vi "Error Handler - Event Handling Loop.vi"(8 "error in (no error)":errorcluster, 10 "Ignore Errors (Runtime)":i32[](array[numeric])) -> (0 "dup error in":errorcluster, 3 "channel":T1)   [LabVIEW 2019]
doc: "Process an error that occurred in the Event Handling Loop, either by ignoring it, or generating an \"Error\" message."
uses:
  Message Queue/Message Cluster.ctl
  03.3 Queued Message Handler/support/Message Queue/Message Queue.lvlib
  <extravilib>/ChannelInstances/Messenger-t'Message Queue.lvlib-Message Cluster.ctl'/))Channel.ctl
  <extravilib>/ChannelInstances/Messenger-t'Message Queue.lvlib-Message Cluster.ctl'.lvlib
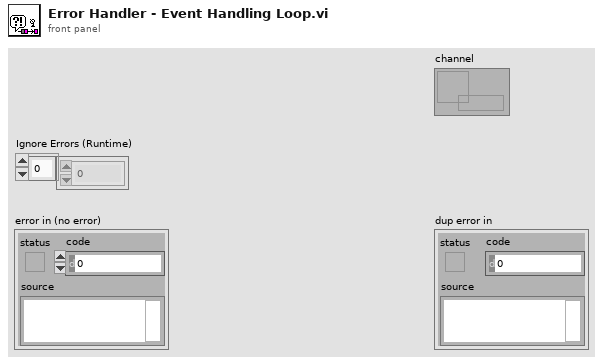
[diagram p1: front panel]
types:
  T1 = typedef "Messenger-t'Message Queue.lvlib-Message Cluster.ctl'.lvlib/))Channel.ctl" = refnum<queue>
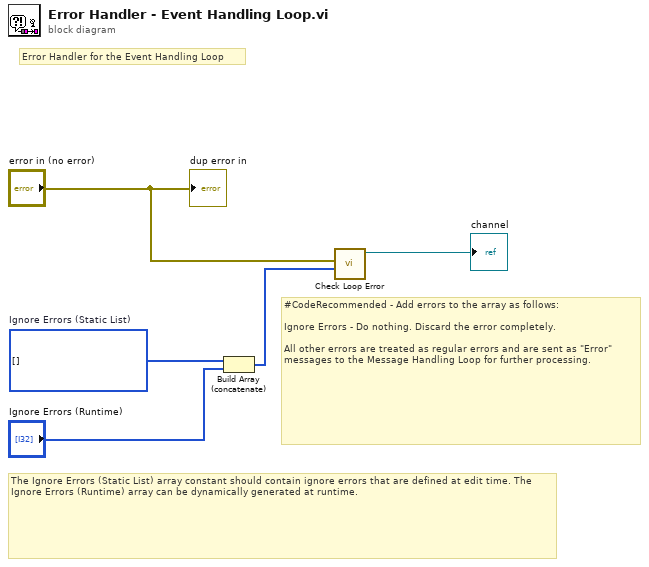
[diagram p0: block diagram]
diagram:
  w5 = i32[] []  # Ignore Errors (Static List)
  # "The Ignore Errors (Static List) array constant should contain ignore errors that are defined at edit time. The Ignore Errors (Runtime) array can be dynamically generated at runtime."
  # "#CodeRecommended - Add errors to the array as follows:\n\nIgnore Errors - Do nothing. Discard the error completely.\n\nAll other errors are treated as regular errors and are sent as \"Error\" messages to the Message Handling Loop for further processing."
  # "Error Handler for the Event Handling Loop"
  n1 = Build Array (concatenate)(w5, "Ignore Errors (Runtime)") -> (w4:i32[])
  n2 = call "Check Loop Error.vi"("Ignore Errors"=w4, "error to process"="error in (no error)") -> ("channel"=→"channel":T1)  [unwired: 8 in, 1 out]
  "dup error in" <- "error in (no error)"
